vi "Get Switch Heat.vi"(8 "error in (no error)":errorcluster, 11 "Instrument.Oxford1820 in":refnum<class "Instrument.Oxford1820.lvclass">) -> (0 "error out":errorcluster, 1 "Heater On?":bool, 2 "Switch Heater Status":string, 3 "Instrument.Oxford1820 out":refnum<class "Instrument.Oxford1820.lvclass">)   [LabVIEW 2016, in "Instrument.Oxford1820.lvclass"]
uses:
  Instrument.Oxford1820.lvclass
  Typedefs/Instrument.Oxford1820.Commands-enum.ctl
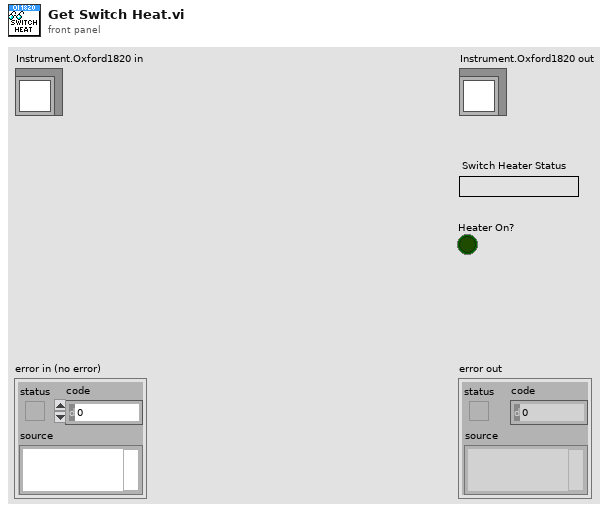
[diagram p1: front panel]
types:
  T1 = typedef "Instrument.Oxford1820.lvclass/Instrument.Oxford1820.Commands-enum.ctl" = enum16{"setAction", "setTarget", "setSwitchHeat", "setLambda", "setFillMode", "setNeedleValve", "setMagnetField", "getStatus", "getTarget", "getSwitchHeat", "getPSUField", "getMagnetField"}
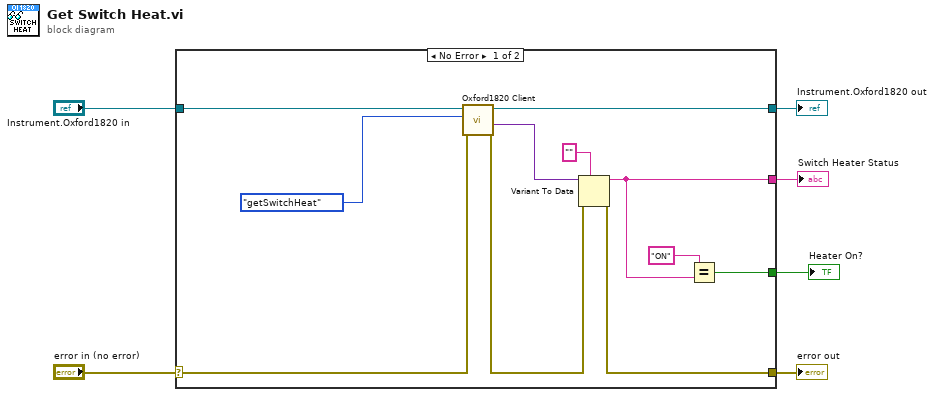
[diagram p0: block diagram]
diagram:
  n1 = case shown="No Error" "error in (no error)" {
    selector: "error in (no error)" -> [w14 w19]
    tunnel: [w11 w19] -> w5
    tunnel: [w15 w18] -> w3
    tunnel: "Instrument.Oxford1820 in" -> [w16 w18]
    tunnel: [w8 _] -> w2
    tunnel: [w7 _] -> w1
    frame No Error {
      n2 = call "Oxford1820 Client.vi"("error in (no error)"=w14, "Commands"=Instrument.Oxford1820.Commands-enum."getSwitchHeat", "Instrument.1820 in"=w16) -> ("error out"=w12:errorcluster, "Data out"=w13:variant, "Instrument.1820 out"=w15:refnum<class "Instrument.Oxford1820.lvclass">)  [unwired: 6 in]
      n3 = Variant To Data(error in=w12, type="", Variant=w13) -> (data=w8:string, error out=w11:errorcluster)
      n4 = Equal?(x="ON", y=w8) -> (x = y?=w7:bool)
    }
    frame Error {
    }
  }
  "error out" <- w5
  "Instrument.Oxford1820 out" <- w3
  "Switch Heater Status" <- w2
  "Heater On?" <- w1
